vi "ztrsm - Solve Linear Eqs (Triangle, multiple) (CDB).vi"(4 "diagonal":T3 items=["Non-unit", "Unit"], 5 "side":T1=1 items=["Left"=1, "Right"=0], 6 "alpha":cdb=1.0+0.0i, 7 "operation A":T5 items=["Direct", "Conjugated & Transposed", "Transposed"], 8 "matrix A type":T4=3 items=["Lower Triangular"=2, "Upper Triangular"=3], 10 "x":T2, 11 "A":T2) -> (0 "error":i32, 3 "ztrsm":T2)   [LabVIEW 2020, in "NI_AALBLAS.lvlib"]
doc: "Solves either op(A)*<B>trsm</B> = <B>alpha</B>*<B>x</B> or <B>trsm</B>*op(A) = <B>alpha</B>*<B>x</B> for <B>trsm</B>."
uses:
  <vilib>/Analysis/NI_AALBLAS.lvlib
  <vilib>/Analysis/Matrix/Datatypes/ComplexMatrix.ctl
  <vilib>/Analysis/BLAS.llb/LV_Transpose.ctl
  <vilib>/Analysis/BLAS.llb/LV_UpLo.ctl
  <vilib>/Analysis/BLAS.llb/LV_Diag.ctl
  <vilib>/Analysis/BLAS.llb/LV_Side.ctl
  <vilib>/Analysis/BLAS.llb/Order.ctl
  <vilib>/Analysis/BLAS.llb/Fucntion.ctl
  <vilib>/Analysis/BLAS.llb/BLAS3 Utility(CDB).vi
  <vilib>/Analysis/Matrix/NI_Matrix.lvlib
panel:
  # "-1"
  # "-1"
  # "ztrsm=alpha*op(A)  *X / ztrsm=alpha*X*op(A)"
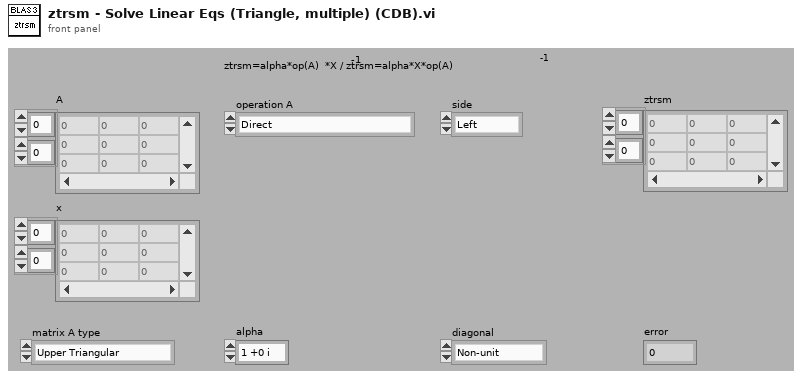
[diagram p1: front panel]
types:
  T1 = typedef "NI_AALBLAS.lvlib/LV_Side.ctl" = i32
  T2 = typedef "NI_Matrix.lvlib/ComplexMatrix.ctl" = cdb[][]
  T3 = typedef "NI_AALBLAS.lvlib/LV_Diag.ctl" = i32
  T4 = typedef "NI_AALBLAS.lvlib/LV_UpLo.ctl" = i32
  T5 = typedef "NI_AALBLAS.lvlib/LV_Transpose.ctl" = i32
  T6 = typedef "NI_AALBLAS.lvlib/Fucntion.ctl" = u16
  T7 = typedef "NI_AALBLAS.lvlib/Order.ctl" = i32
  T8 = typedef "NI_AALBLAS.lvlib/Diag.ctl" = i32
  T9 = typedef "NI_AALBLAS.lvlib/Operation_Transpose.ctl" = i32
  T10 = typedef "NI_AALBLAS.lvlib/UpLo.ctl" = i32
  T11 = typedef "NI_AALBLAS.lvlib/Side.ctl" = i32
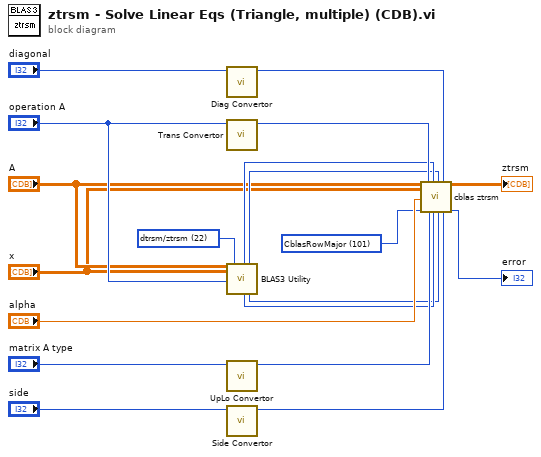
[diagram p0: block diagram]
diagram:
  w1 = T6 22 items=["ddot/zdotu/zdotc", "daxpy/zaxpy", "dnrm2/dznrm2", "dasum/dzasum", "dcopy/zcopy", "dswap/zswap", "drotm", "drot/zdrot", "idamax/izamax", "idamin/izamin", "dgemv/zgemv", "dsymv/zhemv", "dtrmv/ztrmv", "dsyr/zher", "dsyr2/zher2", "dger/zgeru/zgerc", "dtrsv/ztrsv", "dgemm/zgemm", "dsymm/zsymm/zhemm", "dtrmm/ztrmm", "dsyrk/zsyrk/zherk", "dsyr2k/zsyr2k/zher2k", "dtrsm/ztrsm"] ("function")
  w4 = T7 101 items=["CblasRowMajor"=101, "CblasColMajor"=102] ("order")
  n1 = call <vilib>:"Diag Convertor.vi"("diagonal"="diagonal") -> ("diag"=w12:T8)  [unwired: 10 out]
  n2 = call <vilib>:"Trans Convertor.vi"("operation"="operation A") -> ("trans"=w16:T9)  [unwired: 10 out]
  n3 = call-poly <vilib>:"BLAS3 Utility.vi"("A"="A", "B/X"="x", "operation A"="operation A", "function"=w1) -> ("lda"=w7:i32, "m"=w8:i32, "ldb/ldx"=w6:i32, "n"=w5:i32)  [unwired: 2 in, 10 out]
  n4 = call <vilib>:"UpLo Convertor.vi"("triangle matrix type"="matrix A type") -> ("uplo"=w14:T10)  [unwired: 10 out]
  n5 = call <vilib>:"Side Convertor.vi"("LV side"="side") -> ("side"=w10:T11)  [unwired: 10 out]
  n6 = call <vilib>:"cblas ztrsm.vi"("A"="A", "x"="x", "alpha"="alpha", "order"=w4, "transA"=w16, "uplo"=w14, "lda"=w7, "m"=w8, "ldx"=w6, "n"=w5, "diag"=w12, "side"=w10) -> ("ztrsm"=→"ztrsm":T2, "error"=→"error":i32)  [unwired: 6 out]
